vi "Overlay1.vi"   [LabVIEW 2014]
uses:
  QwaveSys_Interface/QwaveSys_Interface.lvlib
  <vilib>/Aledyne-TSXperts/Arduino Compatible Compiler for LabVIEW/Arduino Compatible Compiler for LabVIEW.lvlib
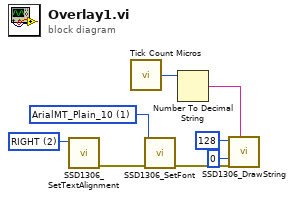
[diagram p0: block diagram]
diagram:
  w6 = u16 1 items=["Calligraffitti_Plain_10", "ArialMT_Plain_10", "ArialMT_Plain_16", "ArialMT_Plain_24"] ("Font")
  w7 = u16 2 items=["LEFT", "CENTER", "RIGHT"] ("alignment")
  n1 = call "SSD1306_SetTextAlignment.vi"("alignment"=w7) -> ("error out"=w8:errorcluster)  [unwired: 10 in]
  n2 = call <vilib>:"Tick Count Micros.vi"() -> ("ticks (us)"=w2:i32)  [unwired: 2 in]
  n3 = call "SSD1306_SetFont.vi"("error in (no error)"=w8, "Font"=w6) -> ("error out"=w5:errorcluster)  [unwired: 9 in]
  n4 = Number To Decimal String(number=w2) -> (decimal integer string=w1:string)  [unwired: 1 in]
  n5 = call "SSD1306_DrawString.vi"("String"=w1, "error in (no error)"=w5, "y"=u8 0, "x"=u8 128) -> ()  [unwired: 7 in, 1 out]
